vi "Get Data Arguments.vi"(8 "error in (no error)":errorcluster, 11 "Connection in":refnum<class "Connection.lvclass">) -> (0 "error out":errorcluster, 3 "Connection out":refnum<class "Connection.lvclass">)   [LabVIEW 2015, in "MDSplus.lvlib" / "Connection.lvclass"]
uses:
  <vilib>/MDSplus_LV2015/Classes/Connection_Class/Connection.lvclass
  <vilib>/MDSplus_LV2015/Classes/Data_Class/Data.lvclass
panel:
  in  "Data Arg4":refnum<class "Data.lvclass">
  in  "Data Arg3":refnum<class "Data.lvclass">
  in  "Data Arg2":refnum<class "Data.lvclass">
  in  "Data Arg1":refnum<class "Data.lvclass">
  in  "Expression in":string
  out "Data out":refnum<class "Data.lvclass">
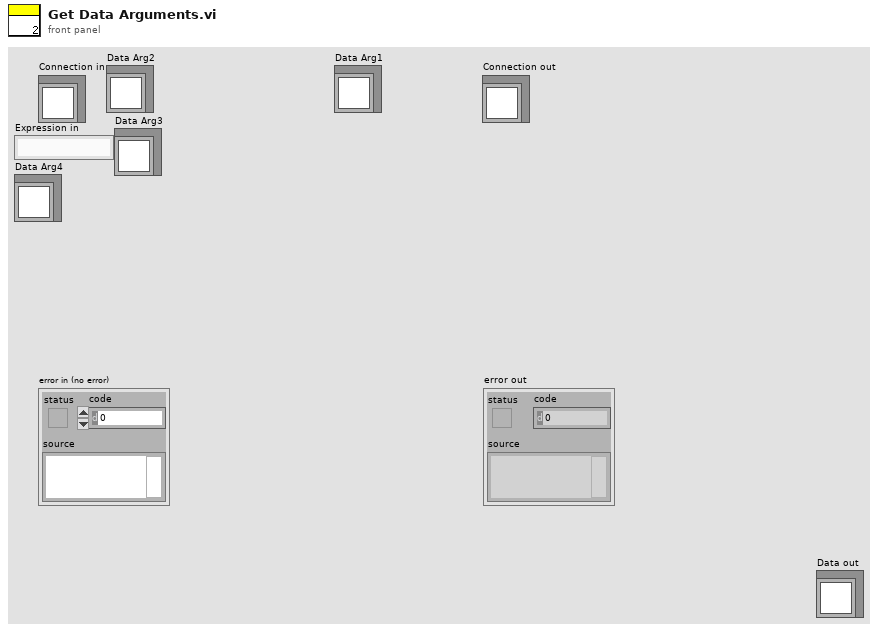
[diagram p1: front panel]
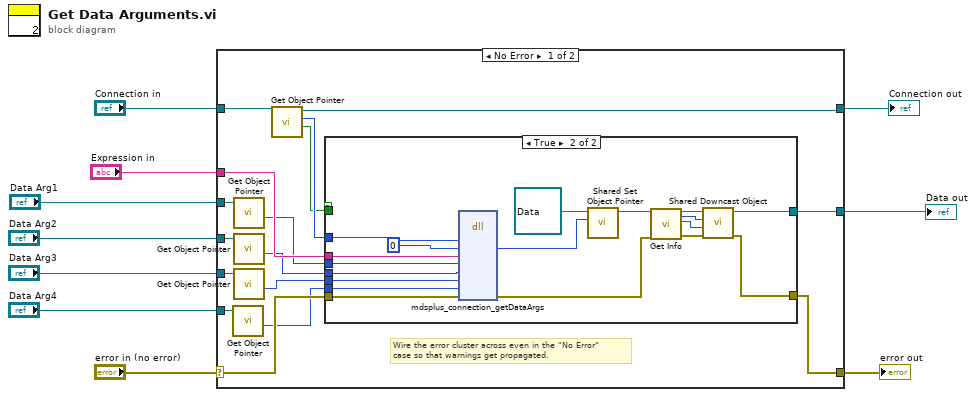
[diagram p0: block diagram]
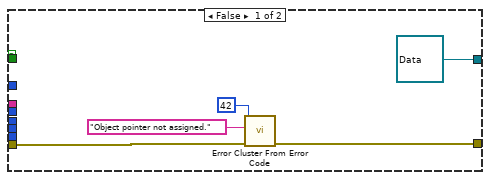
[diagram p2: hidden frame]
diagram:
  n1 = case shown="No Error" "error in (no error)" {
    selector: "error in (no error)" -> [w22 w51]
    tunnel: [w21 w51] -> w9
    tunnel: [w25 w50] -> w7
    tunnel: "Connection in" -> [w26 w50]
    tunnel: [w20 _] -> w6
    tunnel: "Expression in" -> [w19 _]
    tunnel: "Data Arg1" -> [w18 _]
    tunnel: "Data Arg2" -> [w17 _]
    tunnel: "Data Arg3" -> [w16 _]
    tunnel: "Data Arg4" -> [w15 _]
    frame No Error {
      # "Wire the error cluster across even in the \"No Error\"\ncase so that warnings get propagated."
      n2 = call-dynamic <vilib>:"Get Object Pointer.vi"("Data in"=w15) -> ("Object Pointer"=w11:i64)  [unwired: 8 in, 2 out]
      n3 = call-dynamic <vilib>:"Get Object Pointer.vi"("Data in"=w18) -> ("Object Pointer"=w14:i64)  [unwired: 8 in, 2 out]
      n4 = call-dynamic <vilib>:"Get Object Pointer.vi"("Data in"=w17) -> ("Object Pointer"=w13:i64)  [unwired: 8 in, 2 out]
      n5 = call-dynamic <vilib>:"Get Object Pointer.vi"("Data in"=w16) -> ("Object Pointer"=w12:i64)  [unwired: 8 in, 2 out]
      n6 = call <vilib>:"Get Object Pointer.vi"("Connection in"=w26) -> ("Assigned object pointer?"=w23:bool, "Object Pointer"=w24:i64, "Connection out"=w25:refnum<class "Connection.lvclass">)  [unwired: 7 in, 1 out]
      n7 = case shown="True" {
        selector: _ -> [_ _]
        tunnel: [refnum<class "Data.lvclass"> refnum ("Data out") w41] -> w20
        tunnel: w24 -> [_ w40]
        tunnel: w22 -> [w28 w38]
        tunnel: [w27 w37] -> w21
        tunnel: w19 -> [_ w36]
        tunnel: w23 -> [_ _]
        tunnel: w14 -> [_ w35]
        tunnel: w13 -> [_ w34]
        tunnel: w12 -> [_ w33]
        tunnel: w11 -> [_ w32]
        frame False {
          n8 = call <vilib>:"Error Cluster From Error Code.vi"("error in (no error)"=w28, "error message (\"\")"="Object pointer not assigned." ("error message (\"\")"), "error code (0)"=42) -> ("error out"=w27:errorcluster)  [unwired: 6 in]
        }
        frame True {
          n9 = dll-call lib="MDSobjectsLVShr" fn="mdsplus_connection_getDataArgs"("lvConnectionPtr"=w40, "lvDataPtrOut"=i64 0, "expressionIn"=w36, "lvArg1PtrIn"=w35, "lvArg2PtrIn"=w34, "lvArg3PtrIn"=w33, "lvArg4PtrIn"=w32, "error"=w38) -> ("lvDataPtrOut"=w47:i64, "error"=w39:errorcluster)  [unwired: 10 in, 2 out]
          n10 = call <vilib>:"Shared Set Object Pointer.vi"("Object Pointer"=w47, "Data in"=refnum<class "Data.lvclass"> refnum ("Data.lvclass")) -> ("Data out"=w46:refnum<class "Data.lvclass">)  [unwired: 9 in]
          n11 = call-dynamic "Get Info.vi"("Data in"=w46, "error in (no error)"=w39) -> ("Data out"=w45:refnum<class "Data.lvclass">, "Class type out"=w44:u8, "Data type out"=w43:u8, "error out"=w42:errorcluster)  [unwired: 12 in, 2 out]
          n12 = call <vilib>:"Shared Downcast Object.vi"("error in (no error)"=w42, "Data Type"=w43, "Class Type"=w44, "Data in"=w45) -> ("error out"=w37:errorcluster, "Data out"=w41:refnum<class "Data.lvclass">)  [unwired: 6 in]
        }
      }
    }
    frame Error {
    }
  }
  "error out" <- w9
  "Connection out" <- w7
  "Data out" <- w6
